vi "Actor Core.vi"(8 "error in":errorcluster, 11 "CS++DSCTrendViewer in":refnum<class "CS++DSCTrendViewer.lvclass">) -> (0 "error out":errorcluster, 3 "Actor out":refnum<class "Actor.lvclass">)   [LabVIEW 2013, in "CS++DSCTrendViewer.lvlib" / "CS++DSCTrendViewer.lvclass"]
doc: "(<B>Filename</B>: Actor Framework.lvlib:Actor.lvclass:Actor Core.vi)\n\nReceives messages to the actor, reacts to them, and initiates any error handling that may shut the actor down.\n\nDescendant classes may override this VI to append parallel tasks for the actor to complete while it handles messages. Overrides use the Call Parent Method node."
uses:
  CS++DSCTrendViewer.lvclass
  <vilib>/ActorFramework/Actor/Actor.lvclass
  CS++DSCTrendViewer.lvclass/CS++DSCTrendViewer.ctl
  Core/Actors/CS++GUIActor/CS++GUIActor.lvclass/CS++GUIActor.ctl
  Core/Actors/CS++BaseActor/CS++BaseActor.lvclass/CS++BaseActor.ctl
  Core/Actors/CS++GUIActor/CS++GUIActor.lvclass
  <vilib>/ActorFramework/Actor/Actor.lvclass/Actor.ctl
  <vilib>/ActorFramework/Message Enqueuer/Message Enqueuer.lvclass/Message Enqueuer.ctl
  <vilib>/ActorFramework/Message Enqueuer/Init from Existing Queue.vi
  <vilib>/ActorFramework/Message Enqueuer/Enqueue.vi
  <vilib>/ActorFramework/Message Priority Queue/Priority Enqueue.vi
  <vilib>/ActorFramework/Message Enqueuer/Message Enqueuer.lvclass
  <vilib>/ActorFramework/Stop Msg/Stop Msg.lvclass
  Core/Actors/CS++BaseActor/CS++BaseActor.lvclass
panel:
  in  "NIHyperTrend":refnum<k7>(container)
  in  "Stop Button":bool
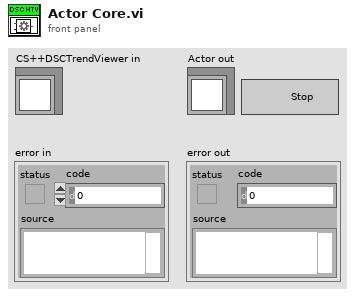
[diagram p1: front panel]
types:
  T1 = enum32{"Invalid", "Standard", "Closed", "Hidden", "Minimized", "Maximized"}
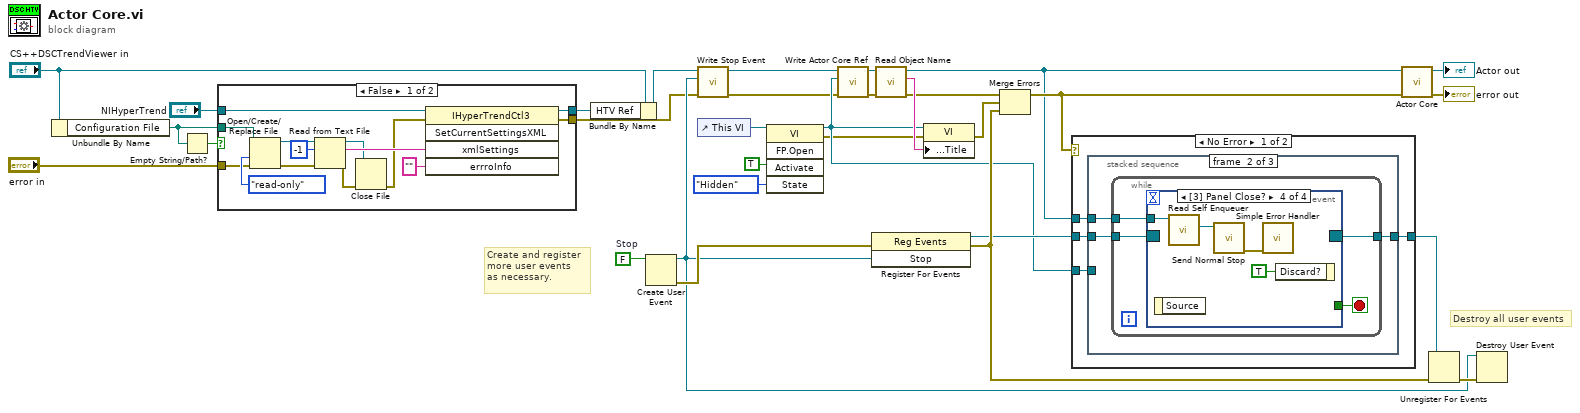
[diagram p0: block diagram]
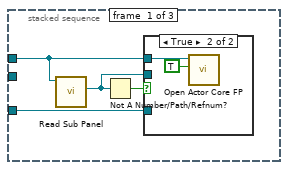
[diagram p3: hidden frame]
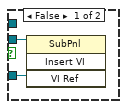
[diagram p4: hidden frame]
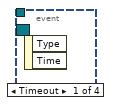
[diagram p5: hidden frame]
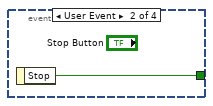
[diagram p6: hidden frame]
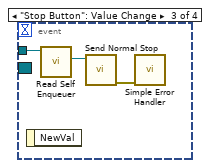
[diagram p7: hidden frame]
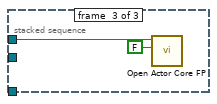
[diagram p8: hidden frame]
diagram:
  w25 = FALSE  # Stop
  # "Destroy all user events"
  # "Create and register \nmore user events\nas necessary."
  n1 = Unbundle By Name("CS++DSCTrendViewer in") -> ("Configuration File"=w5:path)
  n2 = Empty String/Path?(string/path=w5) -> (empty?=w6:bool)
  n3 = case shown="False" w6 {
    tunnel: "NIHyperTrend" -> [w36 w46]
    tunnel: "error in" -> [w35 w47]
    tunnel: [w34 w47] -> w7
    tunnel: w5 -> [w33 _]
    tunnel: [w32 w46] -> w1
    frame False {
      n4 = Open/Create/Replace File(file path (use dialog)=w33, error in=w35, access (0:read/write)=enum16{"read/write", "read-only", "write-only"}."read-only") -> (refnum out=w42:refnum<file>, error out=w43:errorcluster)  [unwired: 3 in, 1 out]
      n5 = Read from Text File(file (use dialog)=w42, count=-1, error in=w43) -> (refnum out=w39:refnum<file>, text=w41:string, error out=w38:errorcluster)  [unwired: 1 in, 1 out]
      n6 = Close File(refnum=w39, error in=w38) -> (error out=w37:errorcluster)  [unwired: 1 out]
      n7 = invoke on="Invoke Node" class="IHyperTrendCtl3" method="SetCurrentSettingsXML"(reference=w36, error in=w37, "xmlSettings"=w41, "errroInfo"="") -> (reference out=w32:refnum<k7>, error out=w34:errorcluster)  [unwired: 1 in, 3 out]
    }
    frame True {
    }
  }
  n8 = Bundle By Name(cluster="CS++DSCTrendViewer in", "HTV Ref"=w1) -> (w2:refnum<class "CS++DSCTrendViewer.lvclass">)
  n9 = Create User Event(user event datatype=w25) -> (user event=w15:refnum<user-event>, error out=w22:errorcluster)  [unwired: 1 in]
  n10 = call "Write Stop Event.vi"("error in (no error)"=w7, "Stop"=w15, "CS++GUIActor in"=w2) -> ("error out"=w13:errorcluster, "CS++GUIActor out"=w14:refnum<class "CS++DSCTrendViewer.lvclass">)  [unwired: 7 in]
  n11 = control-ref of="This VI"() -> (w29:refnum<vi>)
  n12 = invoke class="VI" method="FP.Open"(reference=w29, "Activate"=TRUE ("Activate?"), "State"=T1."Hidden") -> (reference out=w17:refnum<vi>, error out=w16:errorcluster)  [unwired: 2 in, 3 out]
  n13 = call "Write Actor Core Ref.vi"("error in (no error)"=w13, "Actor Core Ref"=w17, "CS++BaseActor in"=w14) -> ("error out"=w12:errorcluster, "CS++BaseActor out"=w11:refnum<class "CS++DSCTrendViewer.lvclass">)  [unwired: 7 in]
  n14 = register-events(error in=w22, w15) -> (reference out=w20:refnum<event-registration>, error out=w21:errorcluster)  [unwired: 1 in]
  n15 = call "Read Object Name.vi"("error in (no error)"=w12, "CS++BaseActor in"=w11) -> ("error out"=w10:errorcluster, "Object Name"=w26:string, "CS++BaseActor out"=w9:refnum<class "CS++DSCTrendViewer.lvclass">)  [unwired: 7 in]
  n16 = property class="VI"(reference=w17, error in=w16, "Front Panel.Title"=w26) -> (error out=w24:errorcluster)  [unwired: 1 out]
  n17 = Merge Errors(w10, w24, w21) -> (w18:errorcluster)
  n18 = case shown="No Error" w18 {
    tunnel: w9 -> [w51 _]
    tunnel: w20 -> [w50 w77]
    tunnel: [w49 w77] -> w19
    tunnel: w17 -> [w48 _]
    frame No Error {
      n19 = stacked-sequence {
        tunnel: w51 -> [w53 w61 w76]
        tunnel: w50 -> [_ w62 _]
        tunnel: [_ w60 _] -> w49
        tunnel: w48 -> [w54 _ _]
        frame #0 {
          n20 = call-dynamic "Read Sub Panel.vi"("CS++GUIActor in"=w53) -> ("Sub Panel"=w52:refnum<vi>)  [unwired: 8 in, 2 out]
          n21 = Not A Number/Path/Refnum?(number/path/refnum=w52) -> (NaN/Path/Refnum?=w55:bool)
          n22 = case shown="True" w55 {
            tunnel: w53 -> [_ w59]
            tunnel: w52 -> [w57 _]
            tunnel: w54 -> [w56 _]
            frame False {
              n23 = invoke class="SubPnl" method="Insert VI"(reference=w57, "VI Ref"=w56) -> ()  [unwired: 2 in, 4 out]
            }
            frame True {
              n24 = call "Open Actor Core FP.vi"("Open FP (F)"=TRUE, "CS++BaseActor in"=w59) -> ()  [unwired: 8 in, 2 out]
            }
          }
        }
        frame #1 {
          n25 = while {
            tunnel: w62 -> [w66]
            tunnel: w61 -> [w65]
            tunnel: [w63] -> w60
            stop <- w64 stop-if-true
            n26 = event shown="[3] Panel Close?" {
              selector: w66 -> [_ _ _ _]
              dyn-events: [_ _ _ _] -> w63
              timeout: _ -> [_ _ _ _]
              tunnel: w65 -> [_ _ w70 w74]
              tunnel: [_ w67 _ _] -> w64
              event Timeout {
                n27 = event-data() -> ()  [unwired: 1 in, 2 out]
              }
              event User Event {
                n28 = event-data() -> ("Stop"=w67:bool)  [unwired: 1 in]
              }
              event "Stop Button": Value Change {
                n29 = event-data() -> ()  [unwired: 1 in, 1 out]
                n30 = call <vilib>:"Read Self Enqueuer.vi"("Actor"=w70) -> ("Self Enqueuer"=w69:refnum<class "Message Enqueuer.lvclass">)  [unwired: 10 in]
                n31 = call <vilib>:"Send Normal Stop.vi"("Message Enqueuer"=w69) -> ("error out"=w68:errorcluster)  [unwired: 10 in]
                n32 = call <vilib>:"Simple Error Handler.vi"("error in (no error)"=w68) -> ()  [unwired: 4 in, 5 out]
              }
              event Panel Close? {
                n33 = event-data() -> ()  [unwired: 1 in, 1 out]
                n34 = call <vilib>:"Read Self Enqueuer.vi"("Actor"=w74) -> ("Self Enqueuer"=w73:refnum<class "Message Enqueuer.lvclass">)  [unwired: 10 in]
                n35 = call <vilib>:"Send Normal Stop.vi"("Message Enqueuer"=w73) -> ("error out"=w72:errorcluster)  [unwired: 10 in]
                n36 = call <vilib>:"Simple Error Handler.vi"("error in (no error)"=w72) -> ()  [unwired: 4 in, 5 out]
                n37 = event-data("Discard?"=TRUE) -> ()  [unwired: 1 in, 1 out]
              }
            }
          }
        }
        frame #2 {
          n38 = call "Open Actor Core FP.vi"("Open FP (F)"=FALSE, "CS++BaseActor in"=w76) -> ()  [unwired: 8 in, 2 out]
        }
      }
    }
    frame Error {
    }
  }
  n39 = call-parent "Actor Core.vi"("error in"=w18, "CS++BaseActor in"=w9) -> ("error out"=→"error out":errorcluster, "Actor out"=→"Actor out":refnum<class "Actor.lvclass">)  [unwired: 8 in]
  n40 = Unregister For Events(event registration refnum=w19, error in=w21) -> (error out=w23:errorcluster)
  n41 = Destroy User Event(user event=w15, error in=w23) -> ()  [unwired: 1 out]
